vi "DrawMarker.vi"(6 "color(black)":u32(colorbox), 7 "Arena Pixel Dim":i32[](array[numeric])=[1000, 512], 8 "Draw An Arrow":bool=TRUE, 10 "Cluster":cluster{"x":dbl, "y":dbl, "angle":dbl}, 11 "picture in":picture) -> (3 "new picture":picture)   [LabVIEW 2015, in "MissionControl2017.lvlib" / "SubVIs - MissionControl2017.lvlib"]
uses:
  SubVIs - MissionControl2017.lvlib
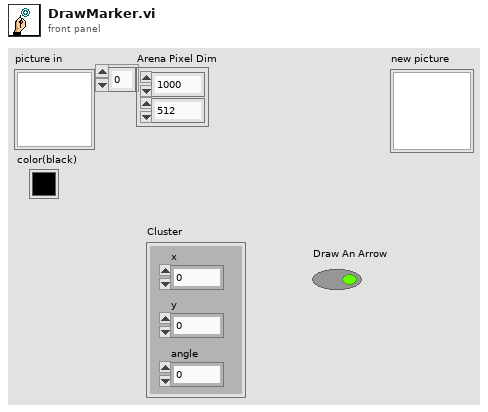
[diagram p1: front panel]
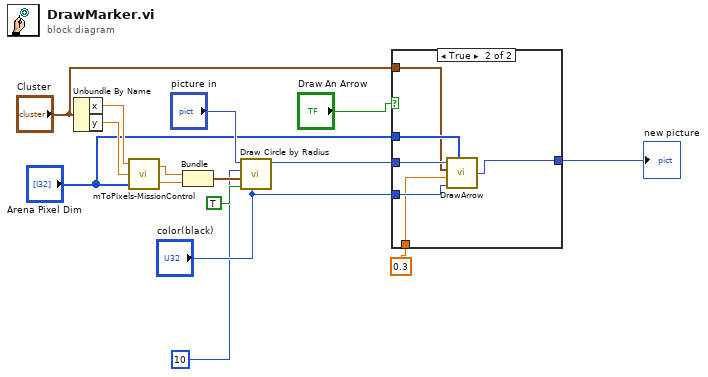
[diagram p0: block diagram]
diagram:
  n1 = Unbundle By Name("Cluster") -> ("x"=w10:dbl, "y"=w9:dbl)
  n2 = call "mToPixels-MissionControl.vi"("Arena Pixel Dim"="Arena Pixel Dim", "y (m)"=w9, "x (m)"=w10) -> ("y (pixels)"=w12:dbl, "x (pixels)"=w13:dbl)
  n3 = Bundle("x (pixels)"=w13, "y (pixels)"=w12) -> (w11:cluster{"x (pixels)":dbl, "y (pixels)":dbl})  [unwired: 1 in]
  n4 = call <vilib>:"Draw Circle by Radius.vi"("color(black)"="color(black)", "fill?(F)"=TRUE, "pixel center"=w11, "radius"=i16 10, "picture"="picture in") -> ("new picture"=w8:picture)  [unwired: 6 in]
  n5 = case shown="True" "Draw An Arrow" {
    tunnel: w8 -> [w16 w22]
    tunnel: [w16 w21] -> w7
    tunnel: "Arena Pixel Dim" -> [_ w20]
    tunnel: "color(black)" -> [_ w19]
    tunnel: 0.3 -> [_ w18]
    tunnel: "Cluster" -> [_ w17]
    frame False {
    }
    frame True {
      n6 = call "DrawArrow.vi"("Arena Pixel Dim"=w20, "Color"=w19, "Length (m)"=w18, "Vector (m)"=w17, "picture"=w22) -> ("new picture"=w21:picture)  [unwired: 1 in]
    }
  }
  "new picture" <- w7
